vi "FileWriter.vi"(10 "Array":dbl[](array[numeric]), 11 "Path in":path) -> (0 "Delimited Conversion Error":errorcluster, 3 "File Error":errorcluster)   [LabVIEW 2023]
uses:
  <vilib>/Analysis/Matrix/NI_Matrix.lvlib
  <vilib>/Analysis/Matrix/Numeric/Conversions/Array To Matrix - RA.vi
  <vilib>/Utility/file.llb/Write Delimited Spreadsheet (DBL).vi
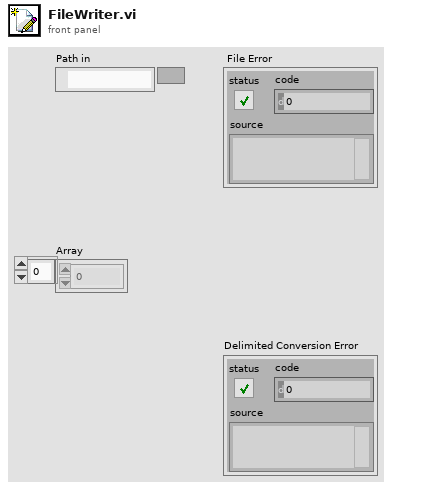
[diagram p1: front panel]
types:
  T1 = typedef "NI_Matrix.lvlib/RealMatrix.ctl" = dbl[][]
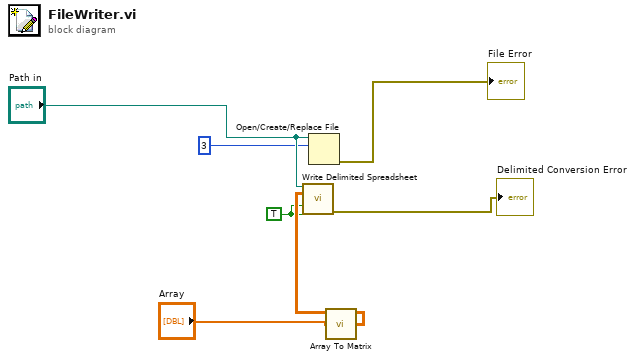
[diagram p0: block diagram]
diagram:
  w4 = TRUE
  n1 = Open/Create/Replace File(file path (use dialog)="Path in", operation (0:open)=3) -> (error out=→"File Error":errorcluster)  [unwired: 4 in, 2 out]
  n2 = call-poly <vilib>:"Array To Matrix.vi"("Real 1D Array"="Array") -> ("Real Matrix (Column Vector)"=w5:T1)
  n3 = call-poly <vilib>:"Write Delimited Spreadsheet.vi"("file path (dialog if empty)"="Path in", "2D data"=w5, "append to file? (new file:F)"=w4, "transpose? (no:F)"=w4) -> ("error out"=→"Delimited Conversion Error":errorcluster)  [unwired: 10 in, 1 out]
